vi "Read Scan Streaming.vi"(8 "error in (no error)":errorcluster, 11 "PF_API in":refnum<class "PF_API.lvclass">) -> (0 "error out":errorcluster, 1 "Distance x Angle":cluster{"Magnitude":dbl, "Phase":dbl}[](array[cluster])=[{"Magnitude"=393.0, "Phase"=0.0}, {"Magnitude"=412.0, "Phase"=-0.25}, {"Magnitude"=398.0, "Phase"=-0.5}, {"Magnitude"=408.0, "Phase"=-0.75}, {"Magnitude"=426.0, "Phase"=-1.0}, {"Magnitude"=419.0, "Phase"=-1.25}, {"Magnitude"=434.0, "Phase"=-1.5}, {"Magnitude"=413.0, "Phase"=-1.75}, {"Magnitude"=425.0, "Phase"=-2.0}, {"Magnitude"=427.0, "Phase"=-2.25}, {"Magnitude"=424.0, "Phase"=-2.5}, {"Magnitude"=415.0, "Phase"=-2.75}, {"Magnitude"=455.0, "Phase"=-3.0}, {"Magnitude"=478.0, "Phase"=-3.25}, {"Magnitude"=541.0, "Phase"=-3.5}, {"Magnitude"=574.0, "Phase"=-3.75}, {"Magnitude"=579.0, "Phase"=-4.0}, {"Magnitude"=601.0, "Phase"=-4.25}, {"Magnitude"=691.0, "Phase"=-4.5}, {"Magnitude"=759.0, "Phase"=-4.75}, {"Magnitude"=794.0, "Phase"=-5.0}, {"Magnitude"=788.0, "Phase"=-5.25}, {"Magnitude"=881.0, "Phase"=-5.5}, {"Magnitude"=882.0, "Phase"=-5.75}, {"Magnitude"=1050.0, "Phase"=-6.0}, {"Magnitude"=954.0, "Phase"=-6.25}, {"Magnitude"=990.0, "Phase"=-6.5}, {"Magnitude"=1198.0, "Phase"=-6.75}, {"Magnitude"=1209.0, "Phase"=-7.0}, {"Magnitude"=1237.0, "Phase"=-7.25}, {"Magnitude"=1231.0, "Phase"=-7.5}, {"Magnitude"=1234.0, "Phase"=-7.75}, {"Magnitude"=1221.0, "Phase"=-8.0}, {"Magnitude"=1213.0, "Phase"=-8.25}, {"Magnitude"=1188.0, "Phase"=-8.5}, {"Magnitude"=1178.0, "Phase"=-8.75}, {"Magnitude"=1174.0, "Phase"=-9.0}, {"Magnitude"=1154.0, "Phase"=-9.25}, {"Magnitude"=1139.0, "Phase"=-9.5}, {"Magnitude"=1024.0, "Phase"=-9.75}, {"Magnitude"=974.0, "Phase"=-10.0}, {"Magnitude"=948.0, "Phase"=-10.25}, {"Magnitude"=913.0, "Phase"=-10.5}, {"Magnitude"=907.0, "Phase"=-10.75}, {"Magnitude"=913.0, "Phase"=-11.0}, {"Magnitude"=919.0, "Phase"=-11.25}, {"Magnitude"=906.0, "Phase"=-11.5}, {"Magnitude"=891.0, "Phase"=-11.75}, {"Magnitude"=844.0, "Phase"=-12.0}, {"Magnitude"=839.0, "Phase"=-12.25}, {"Magnitude"=843.0, "Phase"=-12.5}, {"Magnitude"=838.0, "Phase"=-12.75}, {"Magnitude"=807.0, "Phase"=-13.0}, {"Magnitude"=811.0, "Phase"=-13.25}, {"Magnitude"=798.0, "Phase"=-13.5}, {"Magnitude"=808.0, "Phase"=-13.75}, {"Magnitude"=753.0, "Phase"=-14.0}, {"Magnitude"=708.0, "Phase"=-14.25}, {"Magnitude"=697.0, "Phase"=-14.5}, {"Magnitude"=682.0, "Phase"=-14.75}, {"Magnitude"=684.0, "Phase"=-15.0}, {"Magnitude"=681.0, "Phase"=-15.25}, {"Magnitude"=651.0, "Phase"=-15.5}, {"Magnitude"=665.0, "Phase"=-15.75}, {"Magnitude"=639.0, "Phase"=-16.0}, {"Magnitude"=626.0, "Phase"=-16.25}, {"Magnitude"=635.0, "Phase"=-16.5}, {"Magnitude"=635.0, "Phase"=-16.75}, {"Magnitude"=638.0, "Phase"=-17.0}, {"Magnitude"=625.0, "Phase"=-17.25}, {"Magnitude"=631.0, "Phase"=-17.5}, {"Magnitude"=628.0, "Phase"=-17.75}, {"Magnitude"=619.0, "Phase"=-18.0}, {"Magnitude"=626.0, "Phase"=-18.25}, {"Magnitude"=620.0, "Phase"=-18.5}, {"Magnitude"=622.0, "Phase"=-18.75}, {"Magnitude"=598.0, "Phase"=-19.0}, {"Magnitude"=615.0, "Phase"=-19.25}, {"Magnitude"=601.0, "Phase"=-19.5}, {"Magnitude"=623.0, "Phase"=-19.75}, {"Magnitude"=601.0, "Phase"=-20.0}, {"Magnitude"=605.0, "Phase"=-20.25}, {"Magnitude"=615.0, "Phase"=-20.5}, {"Magnitude"=595.0, "Phase"=-20.75}, {"Magnitude"=585.0, "Phase"=-21.0}, {"Magnitude"=603.0, "Phase"=-21.25}, {"Magnitude"=620.0, "Phase"=-21.5}, {"Magnitude"=602.0, "Phase"=-21.75}, {"Magnitude"=617.0, "Phase"=-22.0}, {"Magnitude"=617.0, "Phase"=-22.25}, {"Magnitude"=600.0, "Phase"=-22.5}, {"Magnitude"=578.0, "Phase"=-22.75}, {"Magnitude"=569.0, "Phase"=-23.0}, {"Magnitude"=553.0, "Phase"=-23.25}, {"Magnitude"=552.0, "Phase"=-23.5}, {"Magnitude"=555.0, "Phase"=-23.75}, {"Magnitude"=540.0, "Phase"=-24.0}, {"Magnitude"=550.0, "Phase"=-24.25}, {"Magnitude"=534.0, "Phase"=-24.5}, {"Magnitude"=530.0, "Phase"=-24.75}, {"Magnitude"=529.0, "Phase"=-25.0}, {"Magnitude"=522.0, "Phase"=-25.25}, {"Magnitude"=538.0, "Phase"=-25.5}, {"Magnitude"=526.0, "Phase"=-25.75}, {"Magnitude"=534.0, "Phase"=-26.0}, {"Magnitude"=518.0, "Phase"=-26.25}, {"Magnitude"=529.0, "Phase"=-26.5}, {"Magnitude"=529.0, "Phase"=-26.75}, {"Magnitude"=509.0, "Phase"=-27.0}, {"Magnitude"=520.0, "Phase"=-27.25}, {"Magnitude"=528.0, "Phase"=-27.5}, {"Magnitude"=522.0, "Phase"=-27.75}, {"Magnitude"=537.0, "Phase"=-28.0}, {"Magnitude"=529.0, "Phase"=-28.25}, {"Magnitude"=517.0, "Phase"=-28.5}, {"Magnitude"=492.0, "Phase"=-28.75}, {"Magnitude"=498.0, "Phase"=-29.0}, {"Magnitude"=442.0, "Phase"=-29.25}, {"Magnitude"=426.0, "Phase"=-29.5}, {"Magnitude"=383.0, "Phase"=-29.75}, {"Magnitude"=314.0, "Phase"=-30.0}, {"Magnitude"=301.0, "Phase"=-30.25}, {"Magnitude"=268.0, "Phase"=-30.5}, {"Magnitude"=191.0, "Phase"=-30.75}, {"Magnitude"=169.0, "Phase"=-31.0}, {"Magnitude"=139.0, "Phase"=-31.25}, {"Magnitude"=125.0, "Phase"=-31.5}, {"Magnitude"=127.0, "Phase"=-31.75}, {"Magnitude"=146.0, "Phase"=-32.0}, {"Magnitude"=117.0, "Phase"=-32.25}, {"Magnitude"=127.0, "Phase"=-32.5}, {"Magnitude"=138.0, "Phase"=-32.75}, {"Magnitude"=162.0, "Phase"=-33.0}, {"Magnitude"=266.0, "Phase"=-33.25}, {"Magnitude"=308.0, "Phase"=-33.5}, {"Magnitude"=355.0, "Phase"=-33.75}, {"Magnitude"=410.0, "Phase"=-34.0}, {"Magnitude"=461.0, "Phase"=-34.25}, {"Magnitude"=480.0, "Phase"=-34.5}, {"Magnitude"=534.0, "Phase"=-34.75}, {"Magnitude"=561.0, "Phase"=-35.0}, {"Magnitude"=560.0, "Phase"=-35.25}, {"Magnitude"=561.0, "Phase"=-35.5}, {"Magnitude"=588.0, "Phase"=-35.75}, {"Magnitude"=582.0, "Phase"=-36.0}, {"Magnitude"=661.0, "Phase"=-36.25}, {"Magnitude"=781.0, "Phase"=-36.5}, {"Magnitude"=1409.0, "Phase"=-36.75}, {"Magnitude"=1416.0, "Phase"=-37.0}, {"Magnitude"=1412.0, "Phase"=-37.25}, {"Magnitude"=1409.0, "Phase"=-37.5}, {"Magnitude"=1414.0, "Phase"=-37.75}, {"Magnitude"=1426.0, "Phase"=-38.0}, {"Magnitude"=1414.0, "Phase"=-38.25}, {"Magnitude"=1399.0, "Phase"=-38.5}, {"Magnitude"=1380.0, "Phase"=-38.75}, {"Magnitude"=1386.0, "Phase"=-39.0}, {"Magnitude"=1412.0, "Phase"=-39.25}, {"Magnitude"=1385.0, "Phase"=-39.5}, {"Magnitude"=1373.0, "Phase"=-39.75}, {"Magnitude"=1375.0, "Phase"=-40.0}, {"Magnitude"=1370.0, "Phase"=-40.25}, {"Magnitude"=1364.0, "Phase"=-40.5}, {"Magnitude"=1360.0, "Phase"=-40.75}, {"Magnitude"=1374.0, "Phase"=-41.0}, {"Magnitude"=1356.0, "Phase"=-41.25}, {"Magnitude"=1357.0, "Phase"=-41.5}, {"Magnitude"=1347.0, "Phase"=-41.75}, {"Magnitude"=1354.0, "Phase"=-42.0}, {"Magnitude"=1351.0, "Phase"=-42.25}, {"Magnitude"=1338.0, "Phase"=-42.5}, {"Magnitude"=1350.0, "Phase"=-42.75}, {"Magnitude"=1341.0, "Phase"=-43.0}, {"Magnitude"=1346.0, "Phase"=-43.25}, {"Magnitude"=1329.0, "Phase"=-43.5}, {"Magnitude"=1321.0, "Phase"=-43.75}, {"Magnitude"=1318.0, "Phase"=-44.0}, {"Magnitude"=1314.0, "Phase"=-44.25}, {"Magnitude"=1307.0, "Phase"=-44.5}, {"Magnitude"=1305.0, "Phase"=-44.75}, {"Magnitude"=1292.0, "Phase"=-45.0}, {"Magnitude"=1314.0, "Phase"=-45.25}, {"Magnitude"=1297.0, "Phase"=-45.5}, {"Magnitude"=1290.0, "Phase"=-45.75}, {"Magnitude"=1294.0, "Phase"=-46.0}, {"Magnitude"=1288.0, "Phase"=-46.25}, {"Magnitude"=1289.0, "Phase"=-46.5}, {"Magnitude"=1267.0, "Phase"=-46.75}, {"Magnitude"=1271.0, "Phase"=-47.0}, {"Magnitude"=1277.0, "Phase"=-47.25}, {"Magnitude"=1279.0, "Phase"=-47.5}, {"Magnitude"=1262.0, "Phase"=-47.75}, {"Magnitude"=1258.0, "Phase"=-48.0}, {"Magnitude"=1261.0, "Phase"=-48.25}, {"Magnitude"=1270.0, "Phase"=-48.5}, {"Magnitude"=1254.0, "Phase"=-48.75}, {"Magnitude"=1262.0, "Phase"=-49.0}, {"Magnitude"=1275.0, "Phase"=-49.25}, {"Magnitude"=1252.0, "Phase"=-49.5}, {"Magnitude"=1264.0, "Phase"=-49.75}, {"Magnitude"=1252.0, "Phase"=-50.0}, {"Magnitude"=1259.0, "Phase"=-50.25}, {"Magnitude"=1242.0, "Phase"=-50.5}, {"Magnitude"=1246.0, "Phase"=-50.75}, {"Magnitude"=1235.0, "Phase"=-51.0}, {"Magnitude"=1246.0, "Phase"=-51.25}, {"Magnitude"=1235.0, "Phase"=-51.5}, {"Magnitude"=1245.0, "Phase"=-51.75}, {"Magnitude"=1222.0, "Phase"=-52.0}, {"Magnitude"=1228.0, "Phase"=-52.25}, {"Magnitude"=1231.0, "Phase"=-52.5}, {"Magnitude"=1227.0, "Phase"=-52.75}, {"Magnitude"=1223.0, "Phase"=-53.0}, {"Magnitude"=1221.0, "Phase"=-53.25}, {"Magnitude"=1236.0, "Phase"=-53.5}, {"Magnitude"=1210.0, "Phase"=-53.75}, {"Magnitude"=1209.0, "Phase"=-54.0}, {"Magnitude"=1200.0, "Phase"=-54.25}, {"Magnitude"=1222.0, "Phase"=-54.5}, {"Magnitude"=1227.0, "Phase"=-54.75}, {"Magnitude"=1203.0, "Phase"=-55.0}, {"Magnitude"=1215.0, "Phase"=-55.25}, {"Magnitude"=1192.0, "Phase"=-55.5}, {"Magnitude"=1208.0, "Phase"=-55.75}, {"Magnitude"=1188.0, "Phase"=-56.0}, {"Magnitude"=1194.0, "Phase"=-56.25}, {"Magnitude"=1182.0, "Phase"=-56.5}, {"Magnitude"=1195.0, "Phase"=-56.75}, {"Magnitude"=1191.0, "Phase"=-57.0}, {"Magnitude"=1181.0, "Phase"=-57.25}, {"Magnitude"=1177.0, "Phase"=-57.5}, {"Magnitude"=1183.0, "Phase"=-57.75}, {"Magnitude"=1206.0, "Phase"=-58.0}, {"Magnitude"=1190.0, "Phase"=-58.25}, {"Magnitude"=1184.0, "Phase"=-58.5}, {"Magnitude"=1182.0, "Phase"=-58.75}, {"Magnitude"=1179.0, "Phase"=-59.0}, {"Magnitude"=1174.0, "Phase"=-59.25}, {"Magnitude"=1186.0, "Phase"=-59.5}, {"Magnitude"=1170.0, "Phase"=-59.75}, {"Magnitude"=1172.0, "Phase"=-60.0}, {"Magnitude"=1172.0, "Phase"=-60.25}, {"Magnitude"=1169.0, "Phase"=-60.5}, {"Magnitude"=1178.0, "Phase"=-60.75}, {"Magnitude"=1183.0, "Phase"=-61.0}, {"Magnitude"=1169.0, "Phase"=-61.25}, {"Magnitude"=1173.0, "Phase"=-61.5}, {"Magnitude"=1179.0, "Phase"=-61.75}, {"Magnitude"=1173.0, "Phase"=-62.0}, {"Magnitude"=1165.0, "Phase"=-62.25}, {"Magnitude"=1165.0, "Phase"=-62.5}, {"Magnitude"=1165.0, "Phase"=-62.75}, {"Magnitude"=1151.0, "Phase"=-63.0}, {"Magnitude"=1157.0, "Phase"=-63.25}, {"Magnitude"=1156.0, "Phase"=-63.5}, {"Magnitude"=1161.0, "Phase"=-63.75}, {"Magnitude"=1173.0, "Phase"=-64.0}, {"Magnitude"=1171.0, "Phase"=-64.25}, {"Magnitude"=1171.0, "Phase"=-64.5}, {"Magnitude"=1152.0, "Phase"=-64.75}, {"Magnitude"=1159.0, "Phase"=-65.0}, {"Magnitude"=1168.0, "Phase"=-65.25}, {"Magnitude"=1160.0, "Phase"=-65.5}, {"Magnitude"=1151.0, "Phase"=-65.75}, {"Magnitude"=1150.0, "Phase"=-66.0}, {"Magnitude"=1151.0, "Phase"=-66.25}, {"Magnitude"=1154.0, "Phase"=-66.5}, {"Magnitude"=1152.0, "Phase"=-66.75}, {"Magnitude"=1146.0, "Phase"=-67.0}, {"Magnitude"=1155.0, "Phase"=-67.25}, {"Magnitude"=1157.0, "Phase"=-67.5}, {"Magnitude"=1145.0, "Phase"=-67.75}, {"Magnitude"=1164.0, "Phase"=-68.0}, {"Magnitude"=1151.0, "Phase"=-68.25}, {"Magnitude"=1149.0, "Phase"=-68.5}, {"Magnitude"=1145.0, "Phase"=-68.75}, {"Magnitude"=1156.0, "Phase"=-69.0}, {"Magnitude"=1155.0, "Phase"=-69.25}, {"Magnitude"=1138.0, "Phase"=-69.5}, {"Magnitude"=1150.0, "Phase"=-69.75}, {"Magnitude"=1150.0, "Phase"=-70.0}, {"Magnitude"=1149.0, "Phase"=-70.25}, {"Magnitude"=1154.0, "Phase"=-70.5}, {"Magnitude"=1161.0, "Phase"=-70.75}, {"Magnitude"=1147.0, "Phase"=-71.0}, {"Magnitude"=1147.0, "Phase"=-71.25}, {"Magnitude"=1150.0, "Phase"=-71.5}, {"Magnitude"=1153.0, "Phase"=-71.75}, {"Magnitude"=1127.0, "Phase"=-72.0}, {"Magnitude"=1162.0, "Phase"=-72.25}, {"Magnitude"=1150.0, "Phase"=-72.5}, {"Magnitude"=1137.0, "Phase"=-72.75}, {"Magnitude"=1135.0, "Phase"=-73.0}, {"Magnitude"=1135.0, "Phase"=-73.25}, {"Magnitude"=1125.0, "Phase"=-73.5}, {"Magnitude"=1133.0, "Phase"=-73.75}, {"Magnitude"=1157.0, "Phase"=-74.0}, {"Magnitude"=1150.0, "Phase"=-74.25}, {"Magnitude"=1142.0, "Phase"=-74.5}, {"Magnitude"=1142.0, "Phase"=-74.75}, {"Magnitude"=1151.0, "Phase"=-75.0}, {"Magnitude"=1150.0, "Phase"=-75.25}, {"Magnitude"=1153.0, "Phase"=-75.5}, {"Magnitude"=1161.0, "Phase"=-75.75}, {"Magnitude"=1154.0, "Phase"=-76.0}, {"Magnitude"=1136.0, "Phase"=-76.25}, {"Magnitude"=1139.0, "Phase"=-76.5}, {"Magnitude"=1143.0, "Phase"=-76.75}, {"Magnitude"=1151.0, "Phase"=-77.0}, {"Magnitude"=1140.0, "Phase"=-77.25}, {"Magnitude"=1151.0, "Phase"=-77.5}, {"Magnitude"=1153.0, "Phase"=-77.75}, {"Magnitude"=1147.0, "Phase"=-78.0}, {"Magnitude"=1141.0, "Phase"=-78.25}, {"Magnitude"=1140.0, "Phase"=-78.5}, {"Magnitude"=1138.0, "Phase"=-78.75}, {"Magnitude"=1142.0, "Phase"=-79.0}, {"Magnitude"=1159.0, "Phase"=-79.25}, {"Magnitude"=1138.0, "Phase"=-79.5}, {"Magnitude"=1167.0, "Phase"=-79.75}, {"Magnitude"=1143.0, "Phase"=-80.0}, {"Magnitude"=1152.0, "Phase"=-80.25}, {"Magnitude"=1137.0, "Phase"=-80.5}, {"Magnitude"=1159.0, "Phase"=-80.75}, {"Magnitude"=1161.0, "Phase"=-81.0}, {"Magnitude"=1156.0, "Phase"=-81.25}, {"Magnitude"=1159.0, "Phase"=-81.5}, {"Magnitude"=1181.0, "Phase"=-81.75}, {"Magnitude"=1160.0, "Phase"=-82.0}, {"Magnitude"=1151.0, "Phase"=-82.25}, {"Magnitude"=1157.0, "Phase"=-82.5}, {"Magnitude"=1156.0, "Phase"=-82.75}, {"Magnitude"=1161.0, "Phase"=-83.0}, {"Magnitude"=1154.0, "Phase"=-83.25}, {"Magnitude"=1149.0, "Phase"=-83.5}, {"Magnitude"=1170.0, "Phase"=-83.75}, {"Magnitude"=1160.0, "Phase"=-84.0}, {"Magnitude"=1150.0, "Phase"=-84.25}, {"Magnitude"=1154.0, "Phase"=-84.5}, {"Magnitude"=1154.0, "Phase"=-84.75}, {"Magnitude"=1164.0, "Phase"=-85.0}, {"Magnitude"=1150.0, "Phase"=-85.25}, {"Magnitude"=1167.0, "Phase"=-85.5}, {"Magnitude"=1168.0, "Phase"=-85.75}, {"Magnitude"=1158.0, "Phase"=-86.0}, {"Magnitude"=1160.0, "Phase"=-86.25}, {"Magnitude"=1171.0, "Phase"=-86.5}, {"Magnitude"=1178.0, "Phase"=-86.75}, {"Magnitude"=1293.0, "Phase"=-87.0}, {"Magnitude"=1785.0, "Phase"=-87.25}, {"Magnitude"=1958.0, "Phase"=-87.5}, {"Magnitude"=1982.0, "Phase"=-87.75}, {"Magnitude"=2005.0, "Phase"=-88.0}, {"Magnitude"=1989.0, "Phase"=-88.25}, {"Magnitude"=1982.0, "Phase"=-88.5}, {"Magnitude"=1979.0, "Phase"=-88.75}, {"Magnitude"=2018.0, "Phase"=-89.0}, {"Magnitude"=2010.0, "Phase"=-89.25}, {"Magnitude"=2000.0, "Phase"=-89.5}, {"Magnitude"=1999.0, "Phase"=-89.75}, {"Magnitude"=2012.0, "Phase"=-90.0}, {"Magnitude"=2029.0, "Phase"=-90.25}, {"Magnitude"=2024.0, "Phase"=-90.5}, {"Magnitude"=2017.0, "Phase"=-90.75}, {"Magnitude"=2029.0, "Phase"=-91.0}, {"Magnitude"=2022.0, "Phase"=-91.25}, {"Magnitude"=2009.0, "Phase"=-91.5}, {"Magnitude"=2020.0, "Phase"=-91.75}, {"Magnitude"=2031.0, "Phase"=-92.0}, {"Magnitude"=2037.0, "Phase"=-92.25}, {"Magnitude"=2029.0, "Phase"=-92.5}, {"Magnitude"=2043.0, "Phase"=-92.75}, {"Magnitude"=2043.0, "Phase"=-93.0}, {"Magnitude"=2053.0, "Phase"=-93.25}, {"Magnitude"=2052.0, "Phase"=-93.5}, {"Magnitude"=2047.0, "Phase"=-93.75}, {"Magnitude"=1991.0, "Phase"=-94.0}, {"Magnitude"=1980.0, "Phase"=-94.25}, {"Magnitude"=1971.0, "Phase"=-94.5}, {"Magnitude"=1952.0, "Phase"=-94.75}, {"Magnitude"=1929.0, "Phase"=-95.0}, {"Magnitude"=1932.0, "Phase"=-95.25}, {"Magnitude"=1920.0, "Phase"=-95.5}, {"Magnitude"=1917.0, "Phase"=-95.75}, {"Magnitude"=1887.0, "Phase"=-96.0}, {"Magnitude"=1888.0, "Phase"=-96.25}, {"Magnitude"=1862.0, "Phase"=-96.5}, {"Magnitude"=1865.0, "Phase"=-96.75}, {"Magnitude"=1851.0, "Phase"=-97.0}, {"Magnitude"=1834.0, "Phase"=-97.25}, {"Magnitude"=1833.0, "Phase"=-97.5}, {"Magnitude"=1814.0, "Phase"=-97.75}, {"Magnitude"=1812.0, "Phase"=-98.0}, {"Magnitude"=1797.0, "Phase"=-98.25}, {"Magnitude"=1799.0, "Phase"=-98.5}, {"Magnitude"=1778.0, "Phase"=-98.75}, {"Magnitude"=1776.0, "Phase"=-99.0}, {"Magnitude"=1756.0, "Phase"=-99.25}, {"Magnitude"=1749.0, "Phase"=-99.5}, {"Magnitude"=1739.0, "Phase"=-99.75}, {"Magnitude"=1725.0, "Phase"=-100.0}, {"Magnitude"=1727.0, "Phase"=-100.25}, {"Magnitude"=1730.0, "Phase"=-100.5}, {"Magnitude"=1704.0, "Phase"=-100.75}, {"Magnitude"=1693.0, "Phase"=-101.0}, {"Magnitude"=1686.0, "Phase"=-101.25}, {"Magnitude"=1674.0, "Phase"=-101.5}, {"Magnitude"=1663.0, "Phase"=-101.75}, {"Magnitude"=1663.0, "Phase"=-102.0}, {"Magnitude"=1658.0, "Phase"=-102.25}, {"Magnitude"=1659.0, "Phase"=-102.5}, {"Magnitude"=1636.0, "Phase"=-102.75}, {"Magnitude"=1636.0, "Phase"=-103.0}, {"Magnitude"=1638.0, "Phase"=-103.25}, {"Magnitude"=1606.0, "Phase"=-103.5}, {"Magnitude"=1611.0, "Phase"=-103.75}, {"Magnitude"=1609.0, "Phase"=-104.0}, {"Magnitude"=1603.0, "Phase"=-104.25}, {"Magnitude"=1587.0, "Phase"=-104.5}, {"Magnitude"=1598.0, "Phase"=-104.75}, {"Magnitude"=1590.0, "Phase"=-105.0}, {"Magnitude"=1575.0, "Phase"=-105.25}, {"Magnitude"=1574.0, "Phase"=-105.5}, {"Magnitude"=1554.0, "Phase"=-105.75}, {"Magnitude"=1558.0, "Phase"=-106.0}, {"Magnitude"=1541.0, "Phase"=-106.25}, {"Magnitude"=1533.0, "Phase"=-106.5}, {"Magnitude"=1538.0, "Phase"=-106.75}, {"Magnitude"=1549.0, "Phase"=-107.0}, {"Magnitude"=1555.0, "Phase"=-107.25}, {"Magnitude"=1551.0, "Phase"=-107.5}, {"Magnitude"=1712.0, "Phase"=-107.75}, {"Magnitude"=1666.0, "Phase"=-108.0}, {"Magnitude"=1538.0, "Phase"=-108.25}, {"Magnitude"=1520.0, "Phase"=-108.5}, {"Magnitude"=1506.0, "Phase"=-108.75}, {"Magnitude"=1497.0, "Phase"=-109.0}, {"Magnitude"=1483.0, "Phase"=-109.25}, {"Magnitude"=1485.0, "Phase"=-109.5}, {"Magnitude"=1467.0, "Phase"=-109.75}, {"Magnitude"=1458.0, "Phase"=-110.0}, {"Magnitude"=1445.0, "Phase"=-110.25}, {"Magnitude"=1451.0, "Phase"=-110.5}, {"Magnitude"=1428.0, "Phase"=-110.75}, {"Magnitude"=1417.0, "Phase"=-111.0}, {"Magnitude"=1425.0, "Phase"=-111.25}, {"Magnitude"=1432.0, "Phase"=-111.5}, {"Magnitude"=1441.0, "Phase"=-111.75}, {"Magnitude"=1432.0, "Phase"=-112.0}, {"Magnitude"=1461.0, "Phase"=-112.25}, {"Magnitude"=1457.0, "Phase"=-112.5}, {"Magnitude"=1465.0, "Phase"=-112.75}, {"Magnitude"=1457.0, "Phase"=-113.0}, {"Magnitude"=1503.0, "Phase"=-113.25}, {"Magnitude"=1496.0, "Phase"=-113.5}, {"Magnitude"=1500.0, "Phase"=-113.75}, {"Magnitude"=1498.0, "Phase"=-114.0}, {"Magnitude"=1508.0, "Phase"=-114.25}, {"Magnitude"=147.0, "Phase"=-114.5}, {"Magnitude"=198.0, "Phase"=-114.75}, {"Magnitude"=474.0, "Phase"=-115.0}, {"Magnitude"=424.0, "Phase"=-115.25}, {"Magnitude"=302.0, "Phase"=-115.5}, {"Magnitude"=220.0, "Phase"=-115.75}, {"Magnitude"=223.0, "Phase"=-116.0}, {"Magnitude"=238.0, "Phase"=-116.25}, {"Magnitude"=224.0, "Phase"=-116.5}, {"Magnitude"=229.0, "Phase"=-116.75}, {"Magnitude"=231.0, "Phase"=-117.0}, {"Magnitude"=222.0, "Phase"=-117.25}, {"Magnitude"=222.0, "Phase"=-117.5}, {"Magnitude"=219.0, "Phase"=-117.75}, {"Magnitude"=237.0, "Phase"=-118.0}, {"Magnitude"=208.0, "Phase"=-118.25}, {"Magnitude"=220.0, "Phase"=-118.5}, {"Magnitude"=223.0, "Phase"=-118.75}, {"Magnitude"=206.0, "Phase"=-119.0}, {"Magnitude"=205.0, "Phase"=-119.25}, {"Magnitude"=201.0, "Phase"=-119.5}, {"Magnitude"=219.0, "Phase"=-119.75}, {"Magnitude"=220.0, "Phase"=-120.0}, {"Magnitude"=215.0, "Phase"=-120.25}, {"Magnitude"=198.0, "Phase"=-120.5}, {"Magnitude"=196.0, "Phase"=-120.75}, {"Magnitude"=207.0, "Phase"=-121.0}, {"Magnitude"=206.0, "Phase"=-121.25}, {"Magnitude"=219.0, "Phase"=-121.5}, {"Magnitude"=200.0, "Phase"=-121.75}, {"Magnitude"=212.0, "Phase"=-122.0}, {"Magnitude"=199.0, "Phase"=-122.25}, {"Magnitude"=202.0, "Phase"=-122.5}, {"Magnitude"=220.0, "Phase"=-122.75}, {"Magnitude"=206.0, "Phase"=-123.0}, {"Magnitude"=210.0, "Phase"=-123.25}, {"Magnitude"=189.0, "Phase"=-123.5}, {"Magnitude"=191.0, "Phase"=-123.75}, {"Magnitude"=211.0, "Phase"=-124.0}, {"Magnitude"=197.0, "Phase"=-124.25}, {"Magnitude"=209.0, "Phase"=-124.5}, {"Magnitude"=213.0, "Phase"=-124.75}, {"Magnitude"=189.0, "Phase"=-125.0}, {"Magnitude"=202.0, "Phase"=-125.25}, {"Magnitude"=177.0, "Phase"=-125.5}, {"Magnitude"=204.0, "Phase"=-125.75}, {"Magnitude"=201.0, "Phase"=-126.0}, {"Magnitude"=197.0, "Phase"=-126.25}, {"Magnitude"=201.0, "Phase"=-126.5}, {"Magnitude"=194.0, "Phase"=-126.75}, {"Magnitude"=177.0, "Phase"=-127.0}, {"Magnitude"=193.0, "Phase"=-127.25}, {"Magnitude"=190.0, "Phase"=-127.5}, {"Magnitude"=191.0, "Phase"=-127.75}, {"Magnitude"=192.0, "Phase"=-128.0}, {"Magnitude"=182.0, "Phase"=-128.25}, {"Magnitude"=192.0, "Phase"=-128.5}, {"Magnitude"=204.0, "Phase"=-128.75}, {"Magnitude"=207.0, "Phase"=-129.0}, {"Magnitude"=205.0, "Phase"=-129.25}, {"Magnitude"=178.0, "Phase"=-129.5}, {"Magnitude"=190.0, "Phase"=-129.75}, {"Magnitude"=192.0, "Phase"=-130.0}, {"Magnitude"=188.0, "Phase"=-130.25}, {"Magnitude"=190.0, "Phase"=-130.5}, {"Magnitude"=184.0, "Phase"=-130.75}, {"Magnitude"=190.0, "Phase"=-131.0}, {"Magnitude"=191.0, "Phase"=-131.25}, {"Magnitude"=197.0, "Phase"=-131.5}, {"Magnitude"=191.0, "Phase"=-131.75}, {"Magnitude"=188.0, "Phase"=-132.0}, {"Magnitude"=198.0, "Phase"=-132.25}, {"Magnitude"=182.0, "Phase"=-132.5}, {"Magnitude"=172.0, "Phase"=-132.75}, {"Magnitude"=173.0, "Phase"=-133.0}, {"Magnitude"=183.0, "Phase"=-133.25}, {"Magnitude"=183.0, "Phase"=-133.5}, {"Magnitude"=177.0, "Phase"=-133.75}, {"Magnitude"=177.0, "Phase"=-134.0}, {"Magnitude"=175.0, "Phase"=-134.25}, {"Magnitude"=180.0, "Phase"=-134.5}, {"Magnitude"=192.0, "Phase"=-134.75}, {"Magnitude"=176.0, "Phase"=-135.0}, {"Magnitude"=185.0, "Phase"=-135.25}, {"Magnitude"=176.0, "Phase"=-135.5}, {"Magnitude"=166.0, "Phase"=-135.75}, {"Magnitude"=177.0, "Phase"=-136.0}, {"Magnitude"=184.0, "Phase"=-136.25}, {"Magnitude"=173.0, "Phase"=-136.5}, {"Magnitude"=178.0, "Phase"=-136.75}, {"Magnitude"=181.0, "Phase"=-137.0}, {"Magnitude"=174.0, "Phase"=-137.25}, {"Magnitude"=186.0, "Phase"=-137.5}, {"Magnitude"=172.0, "Phase"=-137.75}, {"Magnitude"=171.0, "Phase"=-138.0}, {"Magnitude"=180.0, "Phase"=-138.25}, {"Magnitude"=164.0, "Phase"=-138.5}, {"Magnitude"=172.0, "Phase"=-138.75}, {"Magnitude"=169.0, "Phase"=-139.0}, {"Magnitude"=180.0, "Phase"=-139.25}, {"Magnitude"=170.0, "Phase"=-139.5}, {"Magnitude"=176.0, "Phase"=-139.75}, {"Magnitude"=181.0, "Phase"=-140.0}, {"Magnitude"=176.0, "Phase"=-140.25}, {"Magnitude"=164.0, "Phase"=-140.5}, {"Magnitude"=177.0, "Phase"=-140.75}, {"Magnitude"=176.0, "Phase"=-141.0}, {"Magnitude"=167.0, "Phase"=-141.25}, {"Magnitude"=158.0, "Phase"=-141.5}, {"Magnitude"=164.0, "Phase"=-141.75}, {"Magnitude"=165.0, "Phase"=-142.0}, {"Magnitude"=176.0, "Phase"=-142.25}, {"Magnitude"=174.0, "Phase"=-142.5}, {"Magnitude"=172.0, "Phase"=-142.75}, {"Magnitude"=168.0, "Phase"=-143.0}, {"Magnitude"=166.0, "Phase"=-143.25}, {"Magnitude"=166.0, "Phase"=-143.5}, {"Magnitude"=165.0, "Phase"=-143.75}, {"Magnitude"=157.0, "Phase"=-144.0}, {"Magnitude"=165.0, "Phase"=-144.25}, {"Magnitude"=160.0, "Phase"=-144.5}, {"Magnitude"=172.0, "Phase"=-144.75}, {"Magnitude"=164.0, "Phase"=-145.0}, {"Magnitude"=174.0, "Phase"=-145.25}, {"Magnitude"=180.0, "Phase"=-145.5}, {"Magnitude"=167.0, "Phase"=-145.75}, {"Magnitude"=153.0, "Phase"=-146.0}, {"Magnitude"=173.0, "Phase"=-146.25}, {"Magnitude"=156.0, "Phase"=-146.5}, {"Magnitude"=166.0, "Phase"=-146.75}, {"Magnitude"=170.0, "Phase"=-147.0}, {"Magnitude"=162.0, "Phase"=-147.25}, {"Magnitude"=183.0, "Phase"=-147.5}, {"Magnitude"=161.0, "Phase"=-147.75}, {"Magnitude"=163.0, "Phase"=-148.0}, {"Magnitude"=160.0, "Phase"=-148.25}, {"Magnitude"=159.0, "Phase"=-148.5}, {"Magnitude"=152.0, "Phase"=-148.75}, {"Magnitude"=169.0, "Phase"=-149.0}, {"Magnitude"=156.0, "Phase"=-149.25}, {"Magnitude"=159.0, "Phase"=-149.5}, {"Magnitude"=158.0, "Phase"=-149.75}, {"Magnitude"=158.0, "Phase"=-150.0}, {"Magnitude"=147.0, "Phase"=-150.25}, {"Magnitude"=155.0, "Phase"=-150.5}, {"Magnitude"=160.0, "Phase"=-150.75}, {"Magnitude"=159.0, "Phase"=-151.0}, {"Magnitude"=163.0, "Phase"=-151.25}, {"Magnitude"=150.0, "Phase"=-151.5}, {"Magnitude"=162.0, "Phase"=-151.75}, {"Magnitude"=164.0, "Phase"=-152.0}, {"Magnitude"=163.0, "Phase"=-152.25}, {"Magnitude"=159.0, "Phase"=-152.5}, {"Magnitude"=156.0, "Phase"=-152.75}, {"Magnitude"=150.0, "Phase"=-153.0}, {"Magnitude"=172.0, "Phase"=-153.25}, {"Magnitude"=158.0, "Phase"=-153.5}, {"Magnitude"=155.0, "Phase"=-153.75}, {"Magnitude"=157.0, "Phase"=-154.0}, {"Magnitude"=157.0, "Phase"=-154.25}, {"Magnitude"=150.0, "Phase"=-154.5}, {"Magnitude"=157.0, "Phase"=-154.75}, {"Magnitude"=161.0, "Phase"=-155.0}, {"Magnitude"=165.0, "Phase"=-155.25}, {"Magnitude"=156.0, "Phase"=-155.5}, {"Magnitude"=160.0, "Phase"=-155.75}, {"Magnitude"=147.0, "Phase"=-156.0}, {"Magnitude"=148.0, "Phase"=-156.25}, {"Magnitude"=153.0, "Phase"=-156.5}, {"Magnitude"=149.0, "Phase"=-156.75}, {"Magnitude"=160.0, "Phase"=-157.0}, {"Magnitude"=154.0, "Phase"=-157.25}, {"Magnitude"=139.0, "Phase"=-157.5}, {"Magnitude"=161.0, "Phase"=-157.75}, {"Magnitude"=148.0, "Phase"=-158.0}, {"Magnitude"=166.0, "Phase"=-158.25}, {"Magnitude"=146.0, "Phase"=-158.5}, {"Magnitude"=152.0, "Phase"=-158.75}, {"Magnitude"=164.0, "Phase"=-159.0}, {"Magnitude"=165.0, "Phase"=-159.25}, {"Magnitude"=158.0, "Phase"=-159.5}, {"Magnitude"=165.0, "Phase"=-159.75}, {"Magnitude"=168.0, "Phase"=-160.0}, {"Magnitude"=163.0, "Phase"=-160.25}, {"Magnitude"=156.0, "Phase"=-160.5}, {"Magnitude"=166.0, "Phase"=-160.75}, {"Magnitude"=152.0, "Phase"=-161.0}, {"Magnitude"=160.0, "Phase"=-161.25}, {"Magnitude"=163.0, "Phase"=-161.5}, {"Magnitude"=152.0, "Phase"=-161.75}, {"Magnitude"=154.0, "Phase"=-162.0}, {"Magnitude"=150.0, "Phase"=-162.25}, {"Magnitude"=141.0, "Phase"=-162.5}, {"Magnitude"=142.0, "Phase"=-162.75}, {"Magnitude"=144.0, "Phase"=-163.0}, {"Magnitude"=135.0, "Phase"=-163.25}, {"Magnitude"=141.0, "Phase"=-163.5}, {"Magnitude"=155.0, "Phase"=-163.75}, {"Magnitude"=145.0, "Phase"=-164.0}, {"Magnitude"=166.0, "Phase"=-164.25}, {"Magnitude"=157.0, "Phase"=-164.5}, {"Magnitude"=156.0, "Phase"=-164.75}, {"Magnitude"=146.0, "Phase"=-165.0}, {"Magnitude"=152.0, "Phase"=-165.25}, {"Magnitude"=157.0, "Phase"=-165.5}, {"Magnitude"=154.0, "Phase"=-165.75}, {"Magnitude"=151.0, "Phase"=-166.0}, {"Magnitude"=158.0, "Phase"=-166.25}, {"Magnitude"=152.0, "Phase"=-166.5}, {"Magnitude"=153.0, "Phase"=-166.75}, {"Magnitude"=164.0, "Phase"=-167.0}, {"Magnitude"=147.0, "Phase"=-167.25}, {"Magnitude"=149.0, "Phase"=-167.5}, {"Magnitude"=136.0, "Phase"=-167.75}, {"Magnitude"=149.0, "Phase"=-168.0}, {"Magnitude"=156.0, "Phase"=-168.25}, {"Magnitude"=156.0, "Phase"=-168.5}, {"Magnitude"=146.0, "Phase"=-168.75}, {"Magnitude"=134.0, "Phase"=-169.0}, {"Magnitude"=168.0, "Phase"=-169.25}, {"Magnitude"=162.0, "Phase"=-169.5}, {"Magnitude"=156.0, "Phase"=-169.75}, {"Magnitude"=142.0, "Phase"=-170.0}, {"Magnitude"=147.0, "Phase"=-170.25}, {"Magnitude"=158.0, "Phase"=-170.5}, {"Magnitude"=163.0, "Phase"=-170.75}, {"Magnitude"=169.0, "Phase"=-171.0}, {"Magnitude"=150.0, "Phase"=-171.25}, {"Magnitude"=153.0, "Phase"=-171.5}, {"Magnitude"=163.0, "Phase"=-171.75}, {"Magnitude"=164.0, "Phase"=-172.0}, {"Magnitude"=156.0, "Phase"=-172.25}, {"Magnitude"=142.0, "Phase"=-172.5}, {"Magnitude"=146.0, "Phase"=-172.75}, {"Magnitude"=157.0, "Phase"=-173.0}, {"Magnitude"=159.0, "Phase"=-173.25}, {"Magnitude"=172.0, "Phase"=-173.5}, {"Magnitude"=157.0, "Phase"=-173.75}, {"Magnitude"=158.0, "Phase"=-174.0}, {"Magnitude"=169.0, "Phase"=-174.25}, {"Magnitude"=159.0, "Phase"=-174.5}, {"Magnitude"=157.0, "Phase"=-174.75}, {"Magnitude"=155.0, "Phase"=-175.0}, {"Magnitude"=160.0, "Phase"=-175.25}, {"Magnitude"=157.0, "Phase"=-175.5}, {"Magnitude"=154.0, "Phase"=-175.75}, {"Magnitude"=160.0, "Phase"=-176.0}, {"Magnitude"=155.0, "Phase"=-176.25}, {"Magnitude"=154.0, "Phase"=-176.5}, {"Magnitude"=156.0, "Phase"=-176.75}, {"Magnitude"=147.0, "Phase"=-177.0}, {"Magnitude"=169.0, "Phase"=-177.25}, {"Magnitude"=146.0, "Phase"=-177.5}, {"Magnitude"=157.0, "Phase"=-177.75}, {"Magnitude"=149.0, "Phase"=-178.0}, {"Magnitude"=160.0, "Phase"=-178.25}, {"Magnitude"=153.0, "Phase"=-178.5}, {"Magnitude"=146.0, "Phase"=-178.75}, {"Magnitude"=160.0, "Phase"=-179.0}, {"Magnitude"=158.0, "Phase"=-179.25}, {"Magnitude"=174.0, "Phase"=-179.5}, {"Magnitude"=161.0, "Phase"=-179.75}, {"Magnitude"=153.0, "Phase"=-180.0}, {"Magnitude"=152.0, "Phase"=-180.25}, {"Magnitude"=157.0, "Phase"=-180.5}, {"Magnitude"=152.0, "Phase"=-180.75}, {"Magnitude"=161.0, "Phase"=-181.0}, {"Magnitude"=152.0, "Phase"=-181.25}, {"Magnitude"=160.0, "Phase"=-181.5}, {"Magnitude"=145.0, "Phase"=-181.75}, {"Magnitude"=170.0, "Phase"=-182.0}, {"Magnitude"=156.0, "Phase"=-182.25}, {"Magnitude"=173.0, "Phase"=-182.5}, {"Magnitude"=158.0, "Phase"=-182.75}, {"Magnitude"=166.0, "Phase"=-183.0}, {"Magnitude"=168.0, "Phase"=-183.25}, {"Magnitude"=165.0, "Phase"=-183.5}, {"Magnitude"=159.0, "Phase"=-183.75}, {"Magnitude"=166.0, "Phase"=-184.0}, {"Magnitude"=175.0, "Phase"=-184.25}, {"Magnitude"=166.0, "Phase"=-184.5}, {"Magnitude"=170.0, "Phase"=-184.75}, {"Magnitude"=159.0, "Phase"=-185.0}, {"Magnitude"=166.0, "Phase"=-185.25}, {"Magnitude"=160.0, "Phase"=-185.5}, {"Magnitude"=169.0, "Phase"=-185.75}, {"Magnitude"=156.0, "Phase"=-186.0}, {"Magnitude"=177.0, "Phase"=-186.25}, {"Magnitude"=160.0, "Phase"=-186.5}, {"Magnitude"=171.0, "Phase"=-186.75}, {"Magnitude"=152.0, "Phase"=-187.0}, {"Magnitude"=161.0, "Phase"=-187.25}, {"Magnitude"=162.0, "Phase"=-187.5}, {"Magnitude"=164.0, "Phase"=-187.75}, {"Magnitude"=168.0, "Phase"=-188.0}, {"Magnitude"=177.0, "Phase"=-188.25}, {"Magnitude"=175.0, "Phase"=-188.5}, {"Magnitude"=166.0, "Phase"=-188.75}, {"Magnitude"=173.0, "Phase"=-189.0}, {"Magnitude"=176.0, "Phase"=-189.25}, {"Magnitude"=164.0, "Phase"=-189.5}, {"Magnitude"=183.0, "Phase"=-189.75}, {"Magnitude"=182.0, "Phase"=-190.0}, {"Magnitude"=176.0, "Phase"=-190.25}, {"Magnitude"=183.0, "Phase"=-190.5}, {"Magnitude"=177.0, "Phase"=-190.75}, {"Magnitude"=185.0, "Phase"=-191.0}, {"Magnitude"=177.0, "Phase"=-191.25}, {"Magnitude"=181.0, "Phase"=-191.5}, {"Magnitude"=174.0, "Phase"=-191.75}, {"Magnitude"=171.0, "Phase"=-192.0}, {"Magnitude"=175.0, "Phase"=-192.25}, {"Magnitude"=173.0, "Phase"=-192.5}, {"Magnitude"=188.0, "Phase"=-192.75}, {"Magnitude"=193.0, "Phase"=-193.0}, {"Magnitude"=190.0, "Phase"=-193.25}, {"Magnitude"=186.0, "Phase"=-193.5}, {"Magnitude"=185.0, "Phase"=-193.75}, {"Magnitude"=188.0, "Phase"=-194.0}, {"Magnitude"=186.0, "Phase"=-194.25}, {"Magnitude"=183.0, "Phase"=-194.5}, {"Magnitude"=177.0, "Phase"=-194.75}, {"Magnitude"=175.0, "Phase"=-195.0}, {"Magnitude"=179.0, "Phase"=-195.25}, {"Magnitude"=179.0, "Phase"=-195.5}, {"Magnitude"=184.0, "Phase"=-195.75}, {"Magnitude"=177.0, "Phase"=-196.0}, {"Magnitude"=198.0, "Phase"=-196.25}, {"Magnitude"=181.0, "Phase"=-196.5}, {"Magnitude"=185.0, "Phase"=-196.75}, {"Magnitude"=196.0, "Phase"=-197.0}, {"Magnitude"=193.0, "Phase"=-197.25}, {"Magnitude"=191.0, "Phase"=-197.5}, {"Magnitude"=196.0, "Phase"=-197.75}, {"Magnitude"=203.0, "Phase"=-198.0}, {"Magnitude"=199.0, "Phase"=-198.25}, {"Magnitude"=190.0, "Phase"=-198.5}, {"Magnitude"=211.0, "Phase"=-198.75}, {"Magnitude"=183.0, "Phase"=-199.0}, {"Magnitude"=195.0, "Phase"=-199.25}, {"Magnitude"=183.0, "Phase"=-199.5}, {"Magnitude"=193.0, "Phase"=-199.75}, {"Magnitude"=185.0, "Phase"=-200.0}, {"Magnitude"=205.0, "Phase"=-200.25}, {"Magnitude"=200.0, "Phase"=-200.5}, {"Magnitude"=205.0, "Phase"=-200.75}, {"Magnitude"=199.0, "Phase"=-201.0}, {"Magnitude"=214.0, "Phase"=-201.25}, {"Magnitude"=184.0, "Phase"=-201.5}, {"Magnitude"=203.0, "Phase"=-201.75}, {"Magnitude"=200.0, "Phase"=-202.0}, {"Magnitude"=208.0, "Phase"=-202.25}, {"Magnitude"=197.0, "Phase"=-202.5}, {"Magnitude"=216.0, "Phase"=-202.75}, {"Magnitude"=195.0, "Phase"=-203.0}, {"Magnitude"=213.0, "Phase"=-203.25}, {"Magnitude"=210.0, "Phase"=-203.5}, {"Magnitude"=212.0, "Phase"=-203.75}, {"Magnitude"=206.0, "Phase"=-204.0}, {"Magnitude"=207.0, "Phase"=-204.25}, {"Magnitude"=195.0, "Phase"=-204.5}, {"Magnitude"=214.0, "Phase"=-204.75}, {"Magnitude"=208.0, "Phase"=-205.0}, {"Magnitude"=215.0, "Phase"=-205.25}, {"Magnitude"=197.0, "Phase"=-205.5}, {"Magnitude"=205.0, "Phase"=-205.75}, {"Magnitude"=207.0, "Phase"=-206.0}, {"Magnitude"=202.0, "Phase"=-206.25}, {"Magnitude"=223.0, "Phase"=-206.5}, {"Magnitude"=214.0, "Phase"=-206.75}, {"Magnitude"=229.0, "Phase"=-207.0}, {"Magnitude"=231.0, "Phase"=-207.25}, {"Magnitude"=228.0, "Phase"=-207.5}, {"Magnitude"=226.0, "Phase"=-207.75}, {"Magnitude"=213.0, "Phase"=-208.0}, {"Magnitude"=227.0, "Phase"=-208.25}, {"Magnitude"=229.0, "Phase"=-208.5}, {"Magnitude"=218.0, "Phase"=-208.75}, {"Magnitude"=231.0, "Phase"=-209.0}, {"Magnitude"=223.0, "Phase"=-209.25}, {"Magnitude"=223.0, "Phase"=-209.5}, {"Magnitude"=222.0, "Phase"=-209.75}, {"Magnitude"=227.0, "Phase"=-210.0}, {"Magnitude"=228.0, "Phase"=-210.25}, {"Magnitude"=236.0, "Phase"=-210.5}, {"Magnitude"=249.0, "Phase"=-210.75}, {"Magnitude"=232.0, "Phase"=-211.0}, {"Magnitude"=235.0, "Phase"=-211.25}, {"Magnitude"=231.0, "Phase"=-211.5}, {"Magnitude"=225.0, "Phase"=-211.75}, {"Magnitude"=244.0, "Phase"=-212.0}, {"Magnitude"=241.0, "Phase"=-212.25}, {"Magnitude"=247.0, "Phase"=-212.5}, {"Magnitude"=252.0, "Phase"=-212.75}, {"Magnitude"=250.0, "Phase"=-213.0}, {"Magnitude"=250.0, "Phase"=-213.25}, {"Magnitude"=262.0, "Phase"=-213.5}, {"Magnitude"=271.0, "Phase"=-213.75}, {"Magnitude"=234.0, "Phase"=-214.0}, {"Magnitude"=254.0, "Phase"=-214.25}, {"Magnitude"=247.0, "Phase"=-214.5}, {"Magnitude"=268.0, "Phase"=-214.75}, {"Magnitude"=255.0, "Phase"=-215.0}, {"Magnitude"=270.0, "Phase"=-215.25}, {"Magnitude"=277.0, "Phase"=-215.5}, {"Magnitude"=251.0, "Phase"=-215.75}, {"Magnitude"=285.0, "Phase"=-216.0}, {"Magnitude"=255.0, "Phase"=-216.25}, {"Magnitude"=263.0, "Phase"=-216.5}, {"Magnitude"=274.0, "Phase"=-216.75}, {"Magnitude"=268.0, "Phase"=-217.0}, {"Magnitude"=281.0, "Phase"=-217.25}, {"Magnitude"=264.0, "Phase"=-217.5}, {"Magnitude"=280.0, "Phase"=-217.75}, {"Magnitude"=254.0, "Phase"=-218.0}, {"Magnitude"=281.0, "Phase"=-218.25}, {"Magnitude"=292.0, "Phase"=-218.5}, {"Magnitude"=286.0, "Phase"=-218.75}, {"Magnitude"=287.0, "Phase"=-219.0}, {"Magnitude"=285.0, "Phase"=-219.25}, {"Magnitude"=287.0, "Phase"=-219.5}, {"Magnitude"=293.0, "Phase"=-219.75}, {"Magnitude"=295.0, "Phase"=-220.0}, {"Magnitude"=303.0, "Phase"=-220.25}, {"Magnitude"=290.0, "Phase"=-220.5}, {"Magnitude"=308.0, "Phase"=-220.75}, {"Magnitude"=314.0, "Phase"=-221.0}, {"Magnitude"=314.0, "Phase"=-221.25}, {"Magnitude"=302.0, "Phase"=-221.5}, {"Magnitude"=327.0, "Phase"=-221.75}, {"Magnitude"=302.0, "Phase"=-222.0}, {"Magnitude"=298.0, "Phase"=-222.25}, {"Magnitude"=309.0, "Phase"=-222.5}, {"Magnitude"=326.0, "Phase"=-222.75}, {"Magnitude"=308.0, "Phase"=-223.0}, {"Magnitude"=325.0, "Phase"=-223.25}, {"Magnitude"=318.0, "Phase"=-223.5}, {"Magnitude"=322.0, "Phase"=-223.75}, {"Magnitude"=315.0, "Phase"=-224.0}, {"Magnitude"=345.0, "Phase"=-224.25}, {"Magnitude"=339.0, "Phase"=-224.5}, {"Magnitude"=350.0, "Phase"=-224.75}, {"Magnitude"=354.0, "Phase"=-225.0}, {"Magnitude"=347.0, "Phase"=-225.25}, {"Magnitude"=346.0, "Phase"=-225.5}, {"Magnitude"=350.0, "Phase"=-225.75}, {"Magnitude"=344.0, "Phase"=-226.0}, {"Magnitude"=353.0, "Phase"=-226.25}, {"Magnitude"=370.0, "Phase"=-226.5}, {"Magnitude"=347.0, "Phase"=-226.75}, {"Magnitude"=366.0, "Phase"=-227.0}, {"Magnitude"=370.0, "Phase"=-227.25}, {"Magnitude"=383.0, "Phase"=-227.5}, {"Magnitude"=375.0, "Phase"=-227.75}, {"Magnitude"=380.0, "Phase"=-228.0}, {"Magnitude"=371.0, "Phase"=-228.25}, {"Magnitude"=382.0, "Phase"=-228.5}, {"Magnitude"=391.0, "Phase"=-228.75}, {"Magnitude"=386.0, "Phase"=-229.0}, {"Magnitude"=411.0, "Phase"=-229.25}, {"Magnitude"=398.0, "Phase"=-229.5}, {"Magnitude"=385.0, "Phase"=-229.75}, {"Magnitude"=400.0, "Phase"=-230.0}, {"Magnitude"=388.0, "Phase"=-230.25}, {"Magnitude"=402.0, "Phase"=-230.5}, {"Magnitude"=399.0, "Phase"=-230.75}, {"Magnitude"=391.0, "Phase"=-231.0}, {"Magnitude"=390.0, "Phase"=-231.25}, {"Magnitude"=383.0, "Phase"=-231.5}, {"Magnitude"=399.0, "Phase"=-231.75}, {"Magnitude"=383.0, "Phase"=-232.0}, {"Magnitude"=404.0, "Phase"=-232.25}, {"Magnitude"=374.0, "Phase"=-232.5}, {"Magnitude"=395.0, "Phase"=-232.75}, {"Magnitude"=392.0, "Phase"=-233.0}, {"Magnitude"=385.0, "Phase"=-233.25}, {"Magnitude"=386.0, "Phase"=-233.5}, {"Magnitude"=380.0, "Phase"=-233.75}, {"Magnitude"=397.0, "Phase"=-234.0}, {"Magnitude"=379.0, "Phase"=-234.25}, {"Magnitude"=391.0, "Phase"=-234.5}, {"Magnitude"=381.0, "Phase"=-234.75}, {"Magnitude"=377.0, "Phase"=-235.0}, {"Magnitude"=389.0, "Phase"=-235.25}, {"Magnitude"=388.0, "Phase"=-235.5}, {"Magnitude"=376.0, "Phase"=-235.75}, {"Magnitude"=374.0, "Phase"=-236.0}, {"Magnitude"=369.0, "Phase"=-236.25}, {"Magnitude"=386.0, "Phase"=-236.5}, {"Magnitude"=378.0, "Phase"=-236.75}, {"Magnitude"=394.0, "Phase"=-237.0}, {"Magnitude"=362.0, "Phase"=-237.25}, {"Magnitude"=386.0, "Phase"=-237.5}, {"Magnitude"=389.0, "Phase"=-237.75}, {"Magnitude"=384.0, "Phase"=-238.0}, {"Magnitude"=383.0, "Phase"=-238.25}, {"Magnitude"=375.0, "Phase"=-238.5}, {"Magnitude"=382.0, "Phase"=-238.75}, {"Magnitude"=378.0, "Phase"=-239.0}, {"Magnitude"=358.0, "Phase"=-239.25}, {"Magnitude"=372.0, "Phase"=-239.5}, {"Magnitude"=369.0, "Phase"=-239.75}, {"Magnitude"=361.0, "Phase"=-240.0}, {"Magnitude"=376.0, "Phase"=-240.25}, {"Magnitude"=365.0, "Phase"=-240.5}, {"Magnitude"=359.0, "Phase"=-240.75}, {"Magnitude"=364.0, "Phase"=-241.0}, {"Magnitude"=376.0, "Phase"=-241.25}, {"Magnitude"=375.0, "Phase"=-241.5}, {"Magnitude"=361.0, "Phase"=-241.75}, {"Magnitude"=347.0, "Phase"=-242.0}, {"Magnitude"=374.0, "Phase"=-242.25}, {"Magnitude"=367.0, "Phase"=-242.5}, {"Magnitude"=373.0, "Phase"=-242.75}, {"Magnitude"=370.0, "Phase"=-243.0}, {"Magnitude"=361.0, "Phase"=-243.25}, {"Magnitude"=367.0, "Phase"=-243.5}, {"Magnitude"=373.0, "Phase"=-243.75}, {"Magnitude"=362.0, "Phase"=-244.0}, {"Magnitude"=359.0, "Phase"=-244.25}, {"Magnitude"=366.0, "Phase"=-244.5}, {"Magnitude"=358.0, "Phase"=-244.75}, {"Magnitude"=363.0, "Phase"=-245.0}, {"Magnitude"=371.0, "Phase"=-245.25}, {"Magnitude"=376.0, "Phase"=-245.5}, {"Magnitude"=370.0, "Phase"=-245.75}, {"Magnitude"=361.0, "Phase"=-246.0}, {"Magnitude"=372.0, "Phase"=-246.25}, {"Magnitude"=345.0, "Phase"=-246.5}, {"Magnitude"=341.0, "Phase"=-246.75}, {"Magnitude"=356.0, "Phase"=-247.0}, {"Magnitude"=358.0, "Phase"=-247.25}, {"Magnitude"=352.0, "Phase"=-247.5}, {"Magnitude"=372.0, "Phase"=-247.75}, {"Magnitude"=387.0, "Phase"=-248.0}, {"Magnitude"=368.0, "Phase"=-248.25}, {"Magnitude"=379.0, "Phase"=-248.5}, {"Magnitude"=373.0, "Phase"=-248.75}, {"Magnitude"=382.0, "Phase"=-249.0}, {"Magnitude"=363.0, "Phase"=-249.25}, {"Magnitude"=371.0, "Phase"=-249.5}, {"Magnitude"=366.0, "Phase"=-249.75}, {"Magnitude"=363.0, "Phase"=-250.0}, {"Magnitude"=366.0, "Phase"=-250.25}, {"Magnitude"=360.0, "Phase"=-250.5}, {"Magnitude"=351.0, "Phase"=-250.75}, {"Magnitude"=341.0, "Phase"=-251.0}, {"Magnitude"=355.0, "Phase"=-251.25}, {"Magnitude"=347.0, "Phase"=-251.5}, {"Magnitude"=352.0, "Phase"=-251.75}, {"Magnitude"=350.0, "Phase"=108.0}, {"Magnitude"=359.0, "Phase"=107.75}, {"Magnitude"=378.0, "Phase"=107.5}, {"Magnitude"=365.0, "Phase"=107.25}, {"Magnitude"=356.0, "Phase"=107.0}, {"Magnitude"=358.0, "Phase"=106.75}, {"Magnitude"=340.0, "Phase"=106.5}, {"Magnitude"=357.0, "Phase"=106.25}, {"Magnitude"=354.0, "Phase"=106.0}, {"Magnitude"=361.0, "Phase"=105.75}, {"Magnitude"=374.0, "Phase"=105.5}, {"Magnitude"=352.0, "Phase"=105.25}, {"Magnitude"=353.0, "Phase"=105.0}, {"Magnitude"=365.0, "Phase"=104.75}, {"Magnitude"=368.0, "Phase"=104.5}, {"Magnitude"=368.0, "Phase"=104.25}, {"Magnitude"=366.0, "Phase"=104.0}, {"Magnitude"=371.0, "Phase"=103.75}, {"Magnitude"=350.0, "Phase"=103.5}, {"Magnitude"=354.0, "Phase"=103.25}, {"Magnitude"=369.0, "Phase"=103.0}, {"Magnitude"=367.0, "Phase"=102.75}, {"Magnitude"=375.0, "Phase"=102.5}, {"Magnitude"=367.0, "Phase"=102.25}, {"Magnitude"=363.0, "Phase"=102.0}, {"Magnitude"=360.0, "Phase"=101.75}, {"Magnitude"=361.0, "Phase"=101.5}, {"Magnitude"=354.0, "Phase"=101.25}, {"Magnitude"=361.0, "Phase"=101.0}, {"Magnitude"=356.0, "Phase"=100.75}, {"Magnitude"=369.0, "Phase"=100.5}, {"Magnitude"=350.0, "Phase"=100.25}, {"Magnitude"=340.0, "Phase"=100.0}, {"Magnitude"=360.0, "Phase"=99.75}, {"Magnitude"=362.0, "Phase"=99.5}, {"Magnitude"=364.0, "Phase"=99.25}, {"Magnitude"=373.0, "Phase"=99.0}, {"Magnitude"=377.0, "Phase"=98.75}, {"Magnitude"=354.0, "Phase"=98.5}, {"Magnitude"=359.0, "Phase"=98.25}, {"Magnitude"=354.0, "Phase"=98.0}, {"Magnitude"=363.0, "Phase"=97.75}, {"Magnitude"=354.0, "Phase"=97.5}, {"Magnitude"=372.0, "Phase"=97.25}, {"Magnitude"=362.0, "Phase"=97.0}, {"Magnitude"=365.0, "Phase"=96.75}, {"Magnitude"=363.0, "Phase"=96.5}, {"Magnitude"=362.0, "Phase"=96.25}, {"Magnitude"=350.0, "Phase"=96.0}, {"Magnitude"=352.0, "Phase"=95.75}, {"Magnitude"=363.0, "Phase"=95.5}, {"Magnitude"=366.0, "Phase"=95.25}, {"Magnitude"=356.0, "Phase"=95.0}, {"Magnitude"=353.0, "Phase"=94.75}, {"Magnitude"=363.0, "Phase"=94.5}, {"Magnitude"=371.0, "Phase"=94.25}, {"Magnitude"=371.0, "Phase"=94.0}, {"Magnitude"=363.0, "Phase"=93.75}, {"Magnitude"=357.0, "Phase"=93.5}, {"Magnitude"=371.0, "Phase"=93.25}, {"Magnitude"=364.0, "Phase"=93.0}, {"Magnitude"=358.0, "Phase"=92.75}, {"Magnitude"=370.0, "Phase"=92.5}, {"Magnitude"=355.0, "Phase"=92.25}, {"Magnitude"=369.0, "Phase"=92.0}, {"Magnitude"=352.0, "Phase"=91.75}, {"Magnitude"=372.0, "Phase"=91.5}, {"Magnitude"=375.0, "Phase"=91.25}, {"Magnitude"=374.0, "Phase"=91.0}, {"Magnitude"=386.0, "Phase"=90.75}, {"Magnitude"=381.0, "Phase"=90.5}, {"Magnitude"=370.0, "Phase"=90.25}, {"Magnitude"=387.0, "Phase"=90.0}, {"Magnitude"=372.0, "Phase"=89.75}, {"Magnitude"=376.0, "Phase"=89.5}, {"Magnitude"=375.0, "Phase"=89.25}, {"Magnitude"=375.0, "Phase"=89.0}, {"Magnitude"=379.0, "Phase"=88.75}, {"Magnitude"=379.0, "Phase"=88.5}, {"Magnitude"=376.0, "Phase"=88.25}, {"Magnitude"=382.0, "Phase"=88.0}, {"Magnitude"=391.0, "Phase"=87.75}, {"Magnitude"=376.0, "Phase"=87.5}, {"Magnitude"=365.0, "Phase"=87.25}, {"Magnitude"=381.0, "Phase"=87.0}, {"Magnitude"=379.0, "Phase"=86.75}, {"Magnitude"=390.0, "Phase"=86.5}, {"Magnitude"=382.0, "Phase"=86.25}, {"Magnitude"=382.0, "Phase"=86.0}, {"Magnitude"=388.0, "Phase"=85.75}, {"Magnitude"=383.0, "Phase"=85.5}, {"Magnitude"=380.0, "Phase"=85.25}, {"Magnitude"=391.0, "Phase"=85.0}, {"Magnitude"=387.0, "Phase"=84.75}, {"Magnitude"=379.0, "Phase"=84.5}, {"Magnitude"=381.0, "Phase"=84.25}, {"Magnitude"=396.0, "Phase"=84.0}, {"Magnitude"=379.0, "Phase"=83.75}, {"Magnitude"=394.0, "Phase"=83.5}, {"Magnitude"=394.0, "Phase"=83.25}, {"Magnitude"=396.0, "Phase"=83.0}, {"Magnitude"=385.0, "Phase"=82.75}, {"Magnitude"=388.0, "Phase"=82.5}, {"Magnitude"=379.0, "Phase"=82.25}, {"Magnitude"=412.0, "Phase"=82.0}, {"Magnitude"=386.0, "Phase"=81.75}, {"Magnitude"=399.0, "Phase"=81.5}, {"Magnitude"=400.0, "Phase"=81.25}, {"Magnitude"=411.0, "Phase"=81.0}, {"Magnitude"=404.0, "Phase"=80.75}, {"Magnitude"=386.0, "Phase"=80.5}, {"Magnitude"=399.0, "Phase"=80.25}, {"Magnitude"=385.0, "Phase"=80.0}, {"Magnitude"=394.0, "Phase"=79.75}, {"Magnitude"=396.0, "Phase"=79.5}, {"Magnitude"=380.0, "Phase"=79.25}, {"Magnitude"=324.0, "Phase"=79.0}, {"Magnitude"=308.0, "Phase"=78.75}, {"Magnitude"=291.0, "Phase"=78.5}, {"Magnitude"=281.0, "Phase"=78.25}, {"Magnitude"=299.0, "Phase"=78.0}, {"Magnitude"=290.0, "Phase"=77.75}, {"Magnitude"=281.0, "Phase"=77.5}, {"Magnitude"=256.0, "Phase"=77.25}, {"Magnitude"=272.0, "Phase"=77.0}, {"Magnitude"=271.0, "Phase"=76.75}, {"Magnitude"=259.0, "Phase"=76.5}, {"Magnitude"=259.0, "Phase"=76.25}, {"Magnitude"=261.0, "Phase"=76.0}, {"Magnitude"=276.0, "Phase"=75.75}, {"Magnitude"=239.0, "Phase"=75.5}, {"Magnitude"=220.0, "Phase"=75.25}, {"Magnitude"=249.0, "Phase"=75.0}, {"Magnitude"=239.0, "Phase"=74.75}, {"Magnitude"=251.0, "Phase"=74.5}, {"Magnitude"=225.0, "Phase"=74.25}, {"Magnitude"=249.0, "Phase"=74.0}, {"Magnitude"=236.0, "Phase"=73.75}, {"Magnitude"=238.0, "Phase"=73.5}, {"Magnitude"=235.0, "Phase"=73.25}, {"Magnitude"=221.0, "Phase"=73.0}, {"Magnitude"=236.0, "Phase"=72.75}, {"Magnitude"=252.0, "Phase"=72.5}, {"Magnitude"=222.0, "Phase"=72.25}, {"Magnitude"=227.0, "Phase"=72.0}, {"Magnitude"=238.0, "Phase"=71.75}, {"Magnitude"=220.0, "Phase"=71.5}, {"Magnitude"=217.0, "Phase"=71.25}, {"Magnitude"=209.0, "Phase"=71.0}, {"Magnitude"=224.0, "Phase"=70.75}, {"Magnitude"=215.0, "Phase"=70.5}, {"Magnitude"=221.0, "Phase"=70.25}, {"Magnitude"=205.0, "Phase"=70.0}, {"Magnitude"=213.0, "Phase"=69.75}, {"Magnitude"=216.0, "Phase"=69.5}, {"Magnitude"=223.0, "Phase"=69.25}, {"Magnitude"=239.0, "Phase"=69.0}, {"Magnitude"=215.0, "Phase"=68.75}, {"Magnitude"=212.0, "Phase"=68.5}, {"Magnitude"=238.0, "Phase"=68.25}, {"Magnitude"=234.0, "Phase"=68.0}, {"Magnitude"=231.0, "Phase"=67.75}, {"Magnitude"=250.0, "Phase"=67.5}, {"Magnitude"=256.0, "Phase"=67.25}, {"Magnitude"=250.0, "Phase"=67.0}, {"Magnitude"=277.0, "Phase"=66.75}, {"Magnitude"=255.0, "Phase"=66.5}, {"Magnitude"=245.0, "Phase"=66.25}, {"Magnitude"=242.0, "Phase"=66.0}, {"Magnitude"=231.0, "Phase"=65.75}, {"Magnitude"=256.0, "Phase"=65.5}, {"Magnitude"=258.0, "Phase"=65.25}, {"Magnitude"=247.0, "Phase"=65.0}, {"Magnitude"=248.0, "Phase"=64.75}, {"Magnitude"=248.0, "Phase"=64.5}, {"Magnitude"=259.0, "Phase"=64.25}, {"Magnitude"=227.0, "Phase"=64.0}, {"Magnitude"=258.0, "Phase"=63.75}, {"Magnitude"=230.0, "Phase"=63.5}, {"Magnitude"=252.0, "Phase"=63.25}, {"Magnitude"=254.0, "Phase"=63.0}, {"Magnitude"=251.0, "Phase"=62.75}, {"Magnitude"=254.0, "Phase"=62.5}, {"Magnitude"=268.0, "Phase"=62.25}, {"Magnitude"=248.0, "Phase"=62.0}, {"Magnitude"=264.0, "Phase"=61.75}, {"Magnitude"=261.0, "Phase"=61.5}, {"Magnitude"=274.0, "Phase"=61.25}, {"Magnitude"=245.0, "Phase"=61.0}, {"Magnitude"=243.0, "Phase"=60.75}, {"Magnitude"=247.0, "Phase"=60.5}, {"Magnitude"=277.0, "Phase"=60.25}, {"Magnitude"=265.0, "Phase"=60.0}, {"Magnitude"=277.0, "Phase"=59.75}, {"Magnitude"=273.0, "Phase"=59.5}, {"Magnitude"=268.0, "Phase"=59.25}, {"Magnitude"=261.0, "Phase"=59.0}, {"Magnitude"=255.0, "Phase"=58.75}, {"Magnitude"=278.0, "Phase"=58.5}, {"Magnitude"=268.0, "Phase"=58.25}, {"Magnitude"=288.0, "Phase"=58.0}, {"Magnitude"=277.0, "Phase"=57.75}, {"Magnitude"=364.0, "Phase"=57.5}, {"Magnitude"=435.0, "Phase"=57.25}, {"Magnitude"=523.0, "Phase"=57.0}, {"Magnitude"=530.0, "Phase"=56.75}, {"Magnitude"=540.0, "Phase"=56.5}, {"Magnitude"=560.0, "Phase"=56.25}, {"Magnitude"=559.0, "Phase"=56.0}, {"Magnitude"=553.0, "Phase"=55.75}, {"Magnitude"=570.0, "Phase"=55.5}, {"Magnitude"=563.0, "Phase"=55.25}, {"Magnitude"=562.0, "Phase"=55.0}, {"Magnitude"=577.0, "Phase"=54.75}, {"Magnitude"=564.0, "Phase"=54.5}, {"Magnitude"=574.0, "Phase"=54.25}, {"Magnitude"=578.0, "Phase"=54.0}, {"Magnitude"=590.0, "Phase"=53.75}, {"Magnitude"=575.0, "Phase"=53.5}, {"Magnitude"=594.0, "Phase"=53.25}, {"Magnitude"=572.0, "Phase"=53.0}, {"Magnitude"=531.0, "Phase"=52.75}, {"Magnitude"=490.0, "Phase"=52.5}, {"Magnitude"=423.0, "Phase"=52.25}, {"Magnitude"=401.0, "Phase"=52.0}, {"Magnitude"=401.0, "Phase"=51.75}, {"Magnitude"=374.0, "Phase"=51.5}, {"Magnitude"=394.0, "Phase"=51.25}, {"Magnitude"=405.0, "Phase"=51.0}, {"Magnitude"=405.0, "Phase"=50.75}, {"Magnitude"=333.0, "Phase"=50.5}, {"Magnitude"=301.0, "Phase"=50.25}, {"Magnitude"=323.0, "Phase"=50.0}, {"Magnitude"=314.0, "Phase"=49.75}, {"Magnitude"=294.0, "Phase"=49.5}, {"Magnitude"=329.0, "Phase"=49.25}, {"Magnitude"=369.0, "Phase"=49.0}, {"Magnitude"=463.0, "Phase"=48.75}, {"Magnitude"=596.0, "Phase"=48.5}, {"Magnitude"=669.0, "Phase"=48.25}, {"Magnitude"=675.0, "Phase"=48.0}, {"Magnitude"=682.0, "Phase"=47.75}, {"Magnitude"=681.0, "Phase"=47.5}, {"Magnitude"=714.0, "Phase"=47.25}, {"Magnitude"=701.0, "Phase"=47.0}, {"Magnitude"=708.0, "Phase"=46.75}, {"Magnitude"=718.0, "Phase"=46.5}, {"Magnitude"=731.0, "Phase"=46.25}, {"Magnitude"=733.0, "Phase"=46.0}, {"Magnitude"=737.0, "Phase"=45.75}, {"Magnitude"=722.0, "Phase"=45.5}, {"Magnitude"=744.0, "Phase"=45.25}, {"Magnitude"=745.0, "Phase"=45.0}, {"Magnitude"=766.0, "Phase"=44.75}, {"Magnitude"=768.0, "Phase"=44.5}, {"Magnitude"=770.0, "Phase"=44.25}, {"Magnitude"=787.0, "Phase"=44.0}, {"Magnitude"=797.0, "Phase"=43.75}, {"Magnitude"=787.0, "Phase"=43.5}, {"Magnitude"=786.0, "Phase"=43.25}, {"Magnitude"=784.0, "Phase"=43.0}, {"Magnitude"=810.0, "Phase"=42.75}, {"Magnitude"=818.0, "Phase"=42.5}, {"Magnitude"=843.0, "Phase"=42.25}, {"Magnitude"=844.0, "Phase"=42.0}, {"Magnitude"=849.0, "Phase"=41.75}, {"Magnitude"=854.0, "Phase"=41.5}, {"Magnitude"=864.0, "Phase"=41.25}, {"Magnitude"=866.0, "Phase"=41.0}, {"Magnitude"=888.0, "Phase"=40.75}, {"Magnitude"=893.0, "Phase"=40.5}, {"Magnitude"=896.0, "Phase"=40.25}, {"Magnitude"=909.0, "Phase"=40.0}, {"Magnitude"=909.0, "Phase"=39.75}, {"Magnitude"=926.0, "Phase"=39.5}, {"Magnitude"=928.0, "Phase"=39.25}, {"Magnitude"=936.0, "Phase"=39.0}, {"Magnitude"=968.0, "Phase"=38.75}, {"Magnitude"=958.0, "Phase"=38.5}, {"Magnitude"=975.0, "Phase"=38.25}, {"Magnitude"=982.0, "Phase"=38.0}, {"Magnitude"=1005.0, "Phase"=37.75}, {"Magnitude"=1010.0, "Phase"=37.5}, {"Magnitude"=754.0, "Phase"=37.25}, {"Magnitude"=471.0, "Phase"=37.0}, {"Magnitude"=321.0, "Phase"=36.75}, {"Magnitude"=319.0, "Phase"=36.5}, {"Magnitude"=408.0, "Phase"=36.25}, {"Magnitude"=601.0, "Phase"=36.0}, {"Magnitude"=749.0, "Phase"=35.75}, {"Magnitude"=744.0, "Phase"=35.5}, {"Magnitude"=755.0, "Phase"=35.25}, {"Magnitude"=809.0, "Phase"=35.0}, {"Magnitude"=824.0, "Phase"=34.75}, {"Magnitude"=838.0, "Phase"=34.5}, {"Magnitude"=845.0, "Phase"=34.25}, {"Magnitude"=866.0, "Phase"=34.0}, {"Magnitude"=949.0, "Phase"=33.75}, {"Magnitude"=905.0, "Phase"=33.5}, {"Magnitude"=1004.0, "Phase"=33.25}, {"Magnitude"=966.0, "Phase"=33.0}, {"Magnitude"=985.0, "Phase"=32.75}, {"Magnitude"=971.0, "Phase"=32.5}, {"Magnitude"=1004.0, "Phase"=32.25}, {"Magnitude"=1035.0, "Phase"=32.0}, {"Magnitude"=1002.0, "Phase"=31.75}, {"Magnitude"=976.0, "Phase"=31.5}, {"Magnitude"=1061.0, "Phase"=31.25}, {"Magnitude"=1040.0, "Phase"=31.0}, {"Magnitude"=1079.0, "Phase"=30.75}, {"Magnitude"=1104.0, "Phase"=30.5}, {"Magnitude"=1072.0, "Phase"=30.25}, {"Magnitude"=1075.0, "Phase"=30.0}, {"Magnitude"=1106.0, "Phase"=29.75}, {"Magnitude"=1116.0, "Phase"=29.5}, {"Magnitude"=1111.0, "Phase"=29.25}, {"Magnitude"=1118.0, "Phase"=29.0}, {"Magnitude"=1084.0, "Phase"=28.75}, {"Magnitude"=949.0, "Phase"=28.5}, {"Magnitude"=989.0, "Phase"=28.25}, {"Magnitude"=1001.0, "Phase"=28.0}, {"Magnitude"=1008.0, "Phase"=27.75}, {"Magnitude"=999.0, "Phase"=27.5}, {"Magnitude"=1011.0, "Phase"=27.25}, {"Magnitude"=992.0, "Phase"=27.0}, {"Magnitude"=1003.0, "Phase"=26.75}, {"Magnitude"=981.0, "Phase"=26.5}, {"Magnitude"=975.0, "Phase"=26.25}, {"Magnitude"=1009.0, "Phase"=26.0}, {"Magnitude"=1034.0, "Phase"=25.75}, {"Magnitude"=1144.0, "Phase"=25.5}, {"Magnitude"=1170.0, "Phase"=25.25}, {"Magnitude"=1176.0, "Phase"=25.0}, {"Magnitude"=1182.0, "Phase"=24.75}, {"Magnitude"=1106.0, "Phase"=24.5}, {"Magnitude"=1096.0, "Phase"=24.25}, {"Magnitude"=1094.0, "Phase"=24.0}, {"Magnitude"=1091.0, "Phase"=23.75}, {"Magnitude"=1108.0, "Phase"=23.5}, {"Magnitude"=1107.0, "Phase"=23.25}, {"Magnitude"=1143.0, "Phase"=23.0}, {"Magnitude"=1150.0, "Phase"=22.75}, {"Magnitude"=1141.0, "Phase"=22.5}, {"Magnitude"=1134.0, "Phase"=22.25}, {"Magnitude"=1163.0, "Phase"=22.0}, {"Magnitude"=1173.0, "Phase"=21.75}, {"Magnitude"=1180.0, "Phase"=21.5}, {"Magnitude"=1168.0, "Phase"=21.25}, {"Magnitude"=1167.0, "Phase"=21.0}, {"Magnitude"=1149.0, "Phase"=20.75}, {"Magnitude"=1151.0, "Phase"=20.5}, {"Magnitude"=1146.0, "Phase"=20.25}, {"Magnitude"=1154.0, "Phase"=20.0}, {"Magnitude"=1156.0, "Phase"=19.75}, {"Magnitude"=1151.0, "Phase"=19.5}, {"Magnitude"=1168.0, "Phase"=19.25}, {"Magnitude"=1167.0, "Phase"=19.0}, {"Magnitude"=1158.0, "Phase"=18.75}, {"Magnitude"=1152.0, "Phase"=18.5}, {"Magnitude"=1147.0, "Phase"=18.25}, {"Magnitude"=1141.0, "Phase"=18.0}, {"Magnitude"=1147.0, "Phase"=17.75}, {"Magnitude"=1152.0, "Phase"=17.5}, {"Magnitude"=1131.0, "Phase"=17.25}, {"Magnitude"=1142.0, "Phase"=17.0}, {"Magnitude"=1159.0, "Phase"=16.75}, {"Magnitude"=1157.0, "Phase"=16.5}, {"Magnitude"=1150.0, "Phase"=16.25}, {"Magnitude"=1163.0, "Phase"=16.0}, {"Magnitude"=1133.0, "Phase"=15.75}, {"Magnitude"=1137.0, "Phase"=15.5}, {"Magnitude"=1146.0, "Phase"=15.25}, {"Magnitude"=1104.0, "Phase"=15.0}, {"Magnitude"=929.0, "Phase"=14.75}, {"Magnitude"=812.0, "Phase"=14.5}, {"Magnitude"=692.0, "Phase"=14.25}, {"Magnitude"=632.0, "Phase"=14.0}, {"Magnitude"=616.0, "Phase"=13.75}, {"Magnitude"=560.0, "Phase"=13.5}, {"Magnitude"=492.0, "Phase"=13.25}, {"Magnitude"=456.0, "Phase"=13.0}, {"Magnitude"=463.0, "Phase"=12.75}, {"Magnitude"=444.0, "Phase"=12.5}, {"Magnitude"=473.0, "Phase"=12.25}, {"Magnitude"=455.0, "Phase"=12.0}, {"Magnitude"=456.0, "Phase"=11.75}, {"Magnitude"=442.0, "Phase"=11.5}, {"Magnitude"=449.0, "Phase"=11.25}, {"Magnitude"=435.0, "Phase"=11.0}, {"Magnitude"=422.0, "Phase"=10.75}, {"Magnitude"=422.0, "Phase"=10.5}, {"Magnitude"=364.0, "Phase"=10.25}, {"Magnitude"=398.0, "Phase"=10.0}, {"Magnitude"=430.0, "Phase"=9.75}, {"Magnitude"=418.0, "Phase"=9.5}, {"Magnitude"=413.0, "Phase"=9.25}, {"Magnitude"=432.0, "Phase"=9.0}, {"Magnitude"=430.0, "Phase"=8.75}, {"Magnitude"=432.0, "Phase"=8.5}, {"Magnitude"=444.0, "Phase"=8.25}, {"Magnitude"=429.0, "Phase"=8.0}, {"Magnitude"=413.0, "Phase"=7.75}, {"Magnitude"=439.0, "Phase"=7.5}, {"Magnitude"=424.0, "Phase"=7.25}, {"Magnitude"=427.0, "Phase"=7.0}, {"Magnitude"=430.0, "Phase"=6.75}, {"Magnitude"=426.0, "Phase"=6.5}, {"Magnitude"=419.0, "Phase"=6.25}, {"Magnitude"=429.0, "Phase"=6.0}, {"Magnitude"=420.0, "Phase"=5.75}, {"Magnitude"=419.0, "Phase"=5.5}, {"Magnitude"=405.0, "Phase"=5.25}, {"Magnitude"=407.0, "Phase"=5.0}, {"Magnitude"=428.0, "Phase"=4.75}, {"Magnitude"=418.0, "Phase"=4.5}, {"Magnitude"=411.0, "Phase"=4.25}, {"Magnitude"=412.0, "Phase"=4.0}, {"Magnitude"=412.0, "Phase"=3.75}, {"Magnitude"=415.0, "Phase"=3.5}, {"Magnitude"=421.0, "Phase"=3.25}, {"Magnitude"=413.0, "Phase"=3.0}, {"Magnitude"=418.0, "Phase"=2.75}, {"Magnitude"=415.0, "Phase"=2.5}, {"Magnitude"=417.0, "Phase"=2.25}, {"Magnitude"=412.0, "Phase"=2.0}, {"Magnitude"=394.0, "Phase"=1.75}, {"Magnitude"=411.0, "Phase"=1.5}, {"Magnitude"=416.0, "Phase"=1.25}, {"Magnitude"=404.0, "Phase"=1.0}, {"Magnitude"=412.0, "Phase"=0.75}, {"Magnitude"=414.0, "Phase"=0.5}, {"Magnitude"=421.0, "Phase"=0.25}], 3 "PF_API out":refnum<class "PF_API.lvclass">)   [LabVIEW 2019, in "PF_API.lvclass"]
doc: "Reads the UDP stream data from the Scanner and decodes it to a Distance x Angle array of clusters."
uses:
  PF_API.lvclass
  PF_API.lvclass/PF_API.ctl
  Packet Classes/Packet/Packet.lvclass
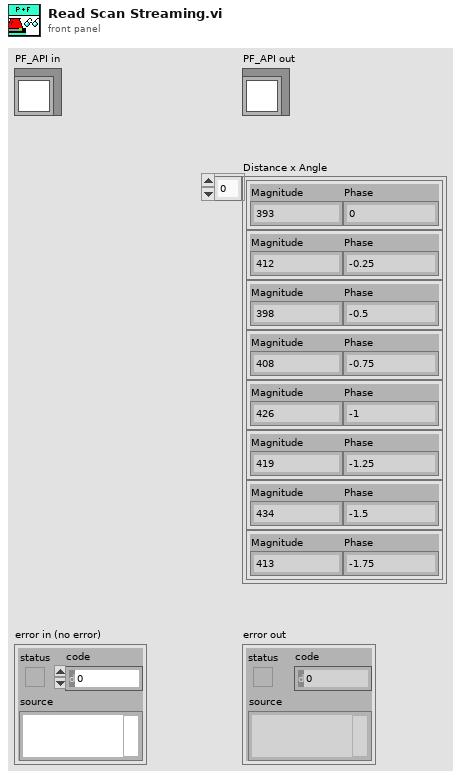
[diagram p1: front panel]
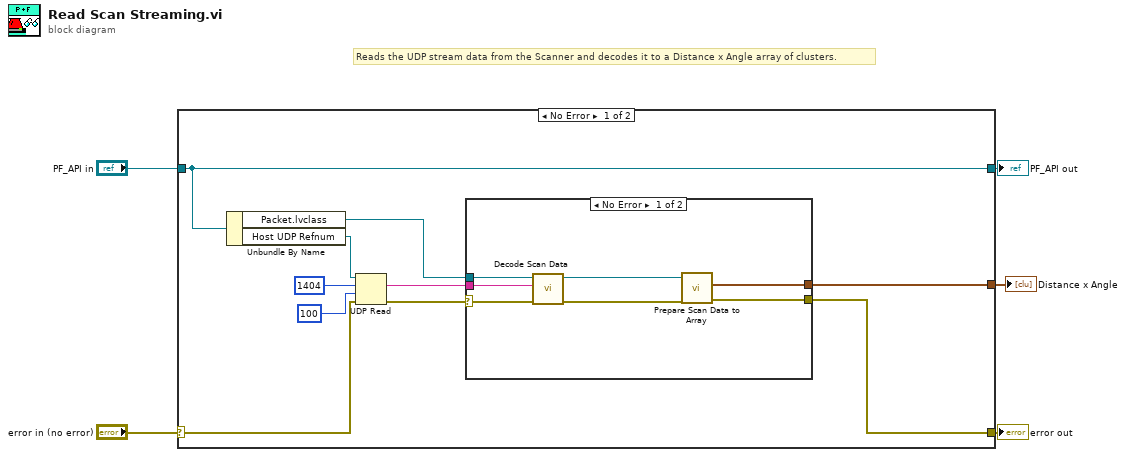
[diagram p0: block diagram]
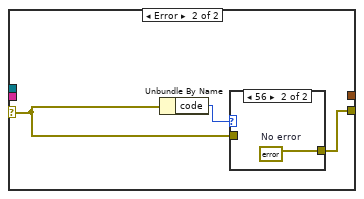
[diagram p2: hidden frame]
diagram:
  # "Reads the UDP stream data from the Scanner and decodes it to a Distance x Angle array of clusters."
  n1 = case shown="No Error" "error in (no error)" {
    selector: "error in (no error)" -> [w8 w29]
    tunnel: [w7 w29] -> w4
    tunnel: [w10 w28] -> w2
    tunnel: "PF_API in" -> [w10 w28]
    tunnel: [w11 _] -> w1
    frame No Error {
      n2 = Unbundle By Name(w10) -> ("Packet.lvclass"=w6:refnum<class "Packet.lvclass">, "Host UDP Refnum"=w9:refnum<k16>)
      n3 = UDP Read(connection ID=w9, max size (548)=1404, timeout ms (25000)=100, 8:w8) -> (data out=w14:string, error out=w13:errorcluster)  [unwired: 3 out]
      n4 = case shown="No Error" w13 {
        selector: w13 -> [w18 w23]
        tunnel: w14 -> [w22 _]
        tunnel: [w17 w24] -> w7
        tunnel: [w20 _] -> w11
        tunnel: w6 -> [w16 _]
        frame No Error {
          # "Sender sent data. Update the chart value."
          n5 = call-dynamic "Decode Scan Data.vi"("error in (no error)"=w18, "Data"=w22, "Packet in"=w16) -> ("error out"=w19:errorcluster, "Packet out"=w21:refnum<class "Packet.lvclass">)  [unwired: 7 in]
          n6 = call-dynamic "Prepare Scan Data to Array.vi"("error in (no error)"=w19, "Packet in"=w21) -> ("error out"=w17:errorcluster, "Distance x Angule"=w20:cluster{"Magnitude":dbl, "Phase":dbl}[])  [unwired: 7 in, 1 out]
        }
        frame Error {
          n7 = Unbundle By Name(w23) -> ("code"=w25:i32)
          n8 = case shown="56" w25 {
            tunnel: [w26 w27] -> w24
            tunnel: w23 -> [w26 _]
            frame Default {
            }
            frame 56 {
              w27 = errorcluster {"status"=FALSE, "code"=0, "source"=""}  # No error
            }
          }
        }
      }
    }
    frame Error {
    }
  }
  "error out" <- w4
  "PF_API out" <- w2
  "Distance x Angle" <- w1
